vi "Plot change of fitting parameters.vi"() -> ()   [LabVIEW 2016]
panel:
  in  "Polynomial Coefficients 2":dbl[][](array[numeric])=[[-6.118000756270661e-11, 5.078581906011179e-10, 3.323766024350423e-09, 4.319320369665537e-08], [-1.05576309639641e-11, 1.4128043416256674e-09, 1.5782151908129023e-10, 6.038454626411456e-09], [-2.8672528691189837e-12, 1.5757035864355753e-09, 2.1483277783334933e-10, 6.478854391491347e-09], [9.772930404589877e-13, 1.6835883057420035e-09, 3.4719771100761e-10, 6.975288437009041e-09], [-5.883264703887976e-12, 1.3657342643288152e-09, 8.278638451974727e-11, 6.036733233138786e-09], [-1.7406101978276473e-11, 1.2767517982489212e-09, 4.820979192165261e-10, 5.90167066932873e-09]] format="%#_6p"
  out "XY Graph":cluster{i32[], dbl[]}[](graph)=[{[0, 1, 2, 3, 4, 5], [3.5148597680894755, 0.6065476909844867, 0.16472687984348436, -0.05614657673950718, 0.3380001284164904, 1.0]}, {[0, 1, 2, 3, 4, 5], [0.397773624676034, 1.1065614660291403, 1.2341502777569373, 1.3186496451785406, 1.0696944121809222, 1.0]}, {[0, 1, 2, 3, 4, 5], [6.8943795271964445, 0.3273640328872844, 0.445620628652539, 0.7201808951423249, 0.1717210990130102, 1.0]}, {[0, 1, 2, 3, 4, 5], [7.318809556950128, 1.0231771585957175, 1.0978000560353645, 1.1819176005973961, 1.0228854796171503, 1.0]}]
  out "size(s)":i32[](array[numeric])=[6, 4]
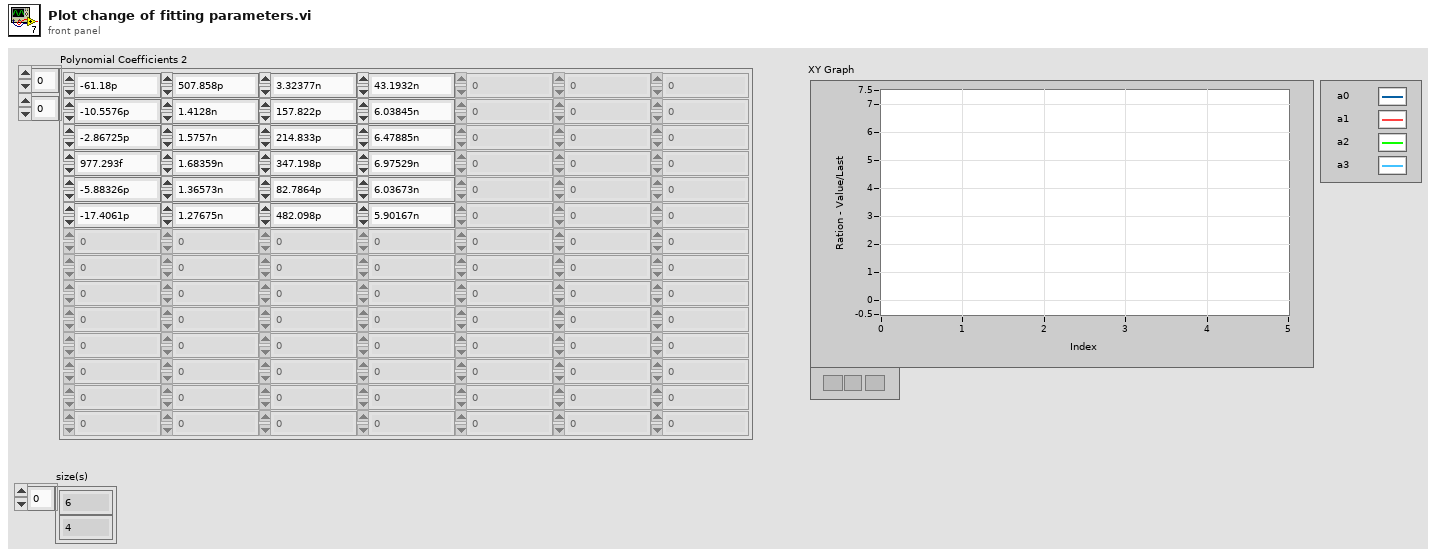
[diagram p1: front panel]
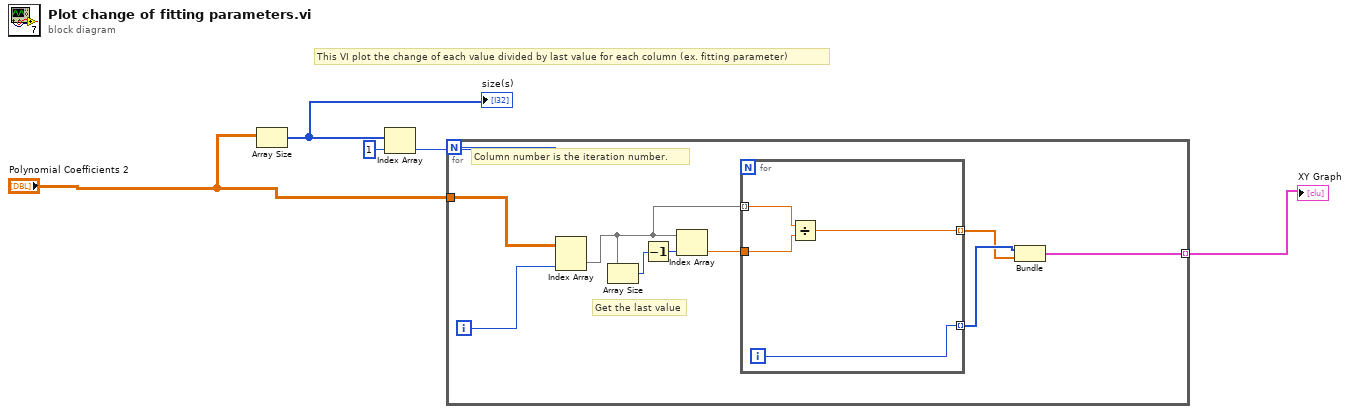
[diagram p0: block diagram]
diagram:
  # "This VI plot the change of each value divided by last value for each column (ex. fitting parameter)"
  n1 = Array Size(array="Polynomial Coefficients 2") -> (size(s)=w5:i32[])
  "size(s)" <- w5
  n2 = Index Array(array=w5, index=1) -> (element=w3:i32)
  n3 = for {
    N: w3 -> [_]
    tunnel: "Polynomial Coefficients 2" -> [w14]
    tunnel: [w8] -> w2 mode=indexing
    i -> [w13]
    # "Column number is the iteration number."
    # "Get the last value"
    n4 = Index Array(array=w14, index (col)=w13) -> (element=w10:dbl[])  [unwired: 1 in]
    n5 = Array Size(array=w10) -> (size(s)=w11:i32)
    n6 = Decrement(x=w11) -> (x-1=w12:i32)
    n7 = Index Array(array=w10, index=w12) -> (element=w9:dbl)
    n8 = for {
      tunnel: w10 -> [w17] mode=indexing
      tunnel: w9 -> [w18]
      tunnel: [w16] -> w6 mode=indexing
      tunnel: [w15] -> w7 mode=indexing
      i -> [w15]
      n9 = Divide(x=w17, y=w18) -> (x/y=w16:dbl)
    }
    n10 = Bundle(w7, w6) -> (w8:cluster{i32[], dbl[]})  [unwired: 1 in]
  }
  "XY Graph" <- w2
